vi "Validate API method.vi"(8 "error in (no error)":errorcluster, 10 "command in":string, 11 "Instrument in":refnum<class "Instrument.lvclass">) -> (0 "error out":errorcluster, 2 "command out":string, 3 "Instrument out":refnum<class "Instrument.lvclass">)   [LabVIEW 2019, in "Instrument.lvclass"]
uses:
  Instrument.lvclass
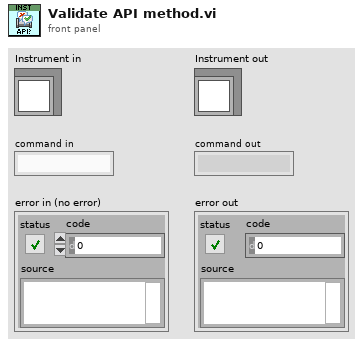
[diagram p1: front panel]
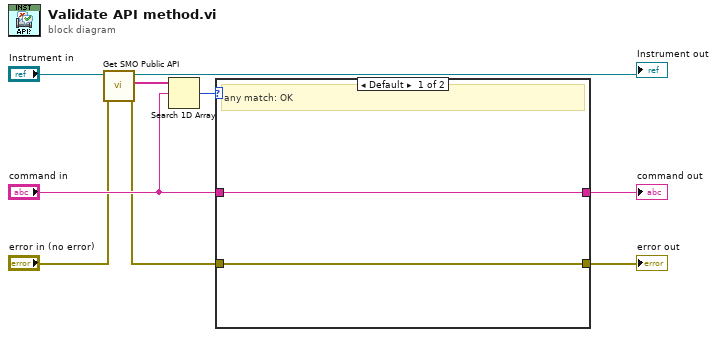
[diagram p0: block diagram]
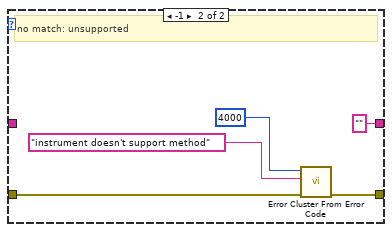
[diagram p2: hidden frame]
diagram:
  n1 = call-dynamic "Get SMO Public API.vi"("error in (no error)"="error in (no error)", "Instrument in"="Instrument in") -> ("error out"=w3:errorcluster, "Commands"=w5:string[], "Instrument out"=→"Instrument out":refnum<class "Instrument.lvclass">)  [unwired: 7 in]
  n2 = Search 1D Array(1D array=w5, element="command in") -> (index of element=w8:i32)  [unwired: 1 in]
  n3 = case shown="Default" w8 {
    tunnel: [w11 w14] -> w9
    tunnel: w3 -> [w11 w13]
    tunnel: [w10 "" ("command in")] -> w7
    tunnel: "command in" -> [w10 _]
    frame Default {
      # "any match: OK"
    }
    frame -1 {
      # "no match: unsupported"
      n4 = call <vilib>:"Error Cluster From Error Code.vi"("error in (no error)"=w13, "error message (\"\")"="instrument doesn't support method" ("error message (\"\")"), "error code (0)"=4000) -> ("error out"=w14:errorcluster)  [unwired: 6 in]
    }
  }
  "error out" <- w9
  "command out" <- w7
